vi "Client_Create.vi"(8 "Error In":errorcluster, 9 "Dinner":refnum<class "DinnerMenu.lvclass">, 10 "Breakfast":refnum<class "BreakfastMenu.lvclass">, 11 "reference in":refnum<class "Client.lvclass">) -> (0 "Error Out":errorcluster, 3 "reference out":refnum<class "Client.lvclass">)   [LabVIEW 2020, in "Client.lvclass"]
uses:
  Client.lvclass
  BreakfastMenu_class/BreakfastMenu.lvclass
  DinnerMenu_class/DinnerMenu.lvclass
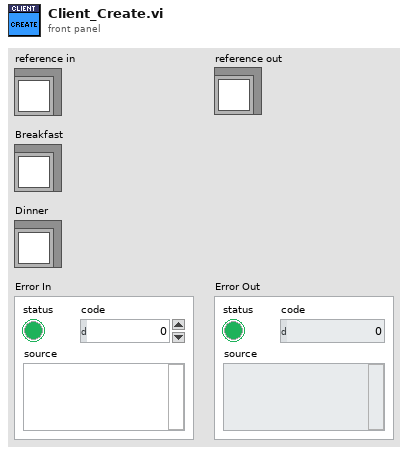
[diagram p1: front panel]
types:
  T1 = typedef "Client.lvclass/ObjectAttributes.ctl" = cluster{"_breakfast":refnum<class "IEnumerable.lvclass">, "_dinner":refnum<class "IEnumerable.lvclass">}
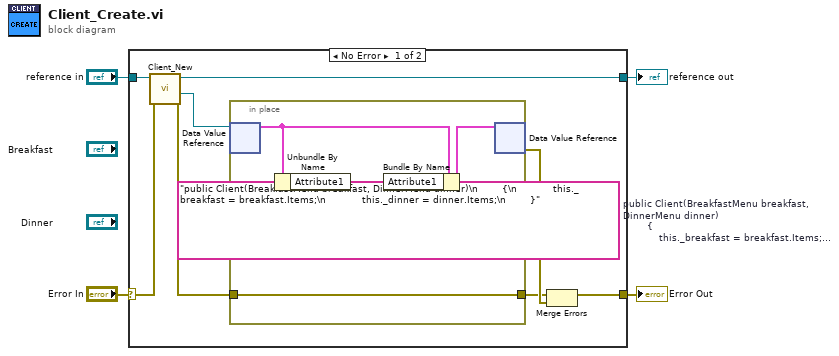
[diagram p0: block diagram]
diagram:
  (unwired) "public Client(BreakfastMenu breakfast, DinnerMenu dinner)\n        {\n            this._breakfast = breakfast.Items;\n            this._dinner = dinner.Items;\n        }"  # public Client(BreakfastMenu breakfast, DinnerMenu dinner)         {             this._breakfast = breakfast.Items;             this._dinner = dinner.Items;         }
  n1 = case shown="No Error" "Error In" {
    selector: "Error In" -> [w11 w18]
    tunnel: [w5 w18] -> w3
    tunnel: "reference in" -> [w12 w17]
    tunnel: [w10 w17] -> w1
    frame No Error {
      n2 = call "Client_New.vi"("error in (no error)"=w11, "reference in"=w12) -> ("error out"=w7:errorcluster, "DVRRefOut"=w8:refnum<data-value>, "reference out"=w10:refnum<class "Client.lvclass">)  [unwired: 6 in, 1 out]
      n3 = in-place {
        in-place-border: w7 -> [w13]
        in-place-border: [w13] -> w6
        n4 = in-place-dvr #1(w8) -> (w15:T1)  [unwired: 1 out]
        n5 = Unbundle By Name(w15) -> ("Attribute1"=w14:dbl)
        n6 = Bundle By Name(cluster=w15, "Attribute1"=w14) -> (w16:T1)
        n7 = in-place-dvr #1(w16) -> (w9:errorcluster)  [unwired: 1 out]
      }
      n8 = Merge Errors(w6, w9) -> (w5:errorcluster)
    }
    frame Error {
      # "VI-TechBaseTemplate_Simple_4x4x4"
    }
  }
  "Error Out" <- w3
  "reference out" <- w1
